vi "myDAQ Errors.vi"(8 "error in (no error)":errorcluster) -> (0 "error out":errorcluster)   [LabVIEW 2012]
doc: "This VI is designed to handel common myDAQ errors and give more useful specific error dialogs. It also finds a control names \"Stop\" in the calling VI and toggels it true to stop the VI."
uses:
  <vilib>/regexp/Match Regular Expression.xnode
panel:
  out "call chain":string[](array[string])
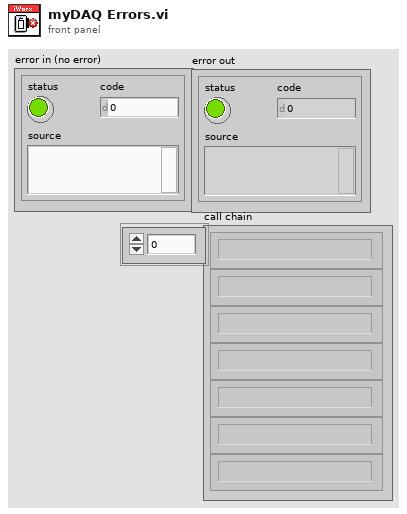
[diagram p1: front panel]
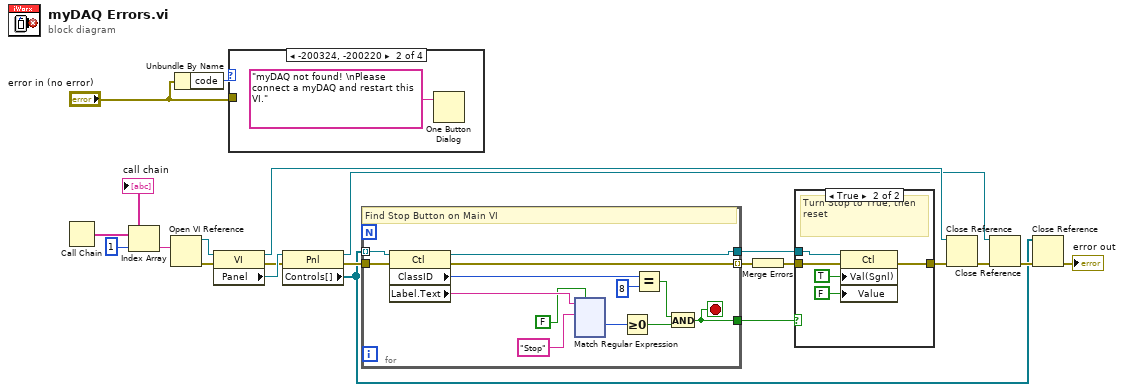
[diagram p0: block diagram]
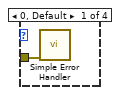
[diagram p3: hidden frame]
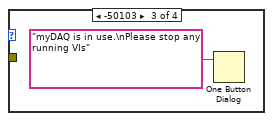
[diagram p4: hidden frame]
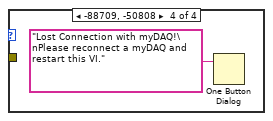
[diagram p5: hidden frame]
diagram:
  n1 = Call Chain() -> (call chain=w20:string[])
  "call chain" <- w20
  n2 = Index Array(array=w20, index=1) -> (element=w18:string)
  n3 = Open VI Reference(vi path=w18) -> (vi reference=w17:refnum<vi>, error out=w16:errorcluster)  [unwired: 5 in]
  n4 = Unbundle By Name("error in (no error)") -> ("code"=w21:i32)
  n5 = property class="VI"(reference=w17, error in=w16) -> (reference out=w8:refnum<vi>, error out=w11:errorcluster, "Panel"=w15:refnum<vi>)
  n6 = case shown="-200324, -200220" w21 {
    tunnel: "error in (no error)" -> [w22 _ _ _]
    frame 0, Default {
      n7 = call <vilib>:"Simple Error Handler.vi"("error in (no error)"=w22) -> ()  [unwired: 4 in, 5 out]
    }
    frame -200324, -200220 {
      n8 = One Button Dialog(message="myDAQ not found! \nPlease connect a myDAQ and restart this VI.") -> ()  [unwired: 1 in, 1 out]
    }
    frame -50103 {
      n9 = One Button Dialog(message="myDAQ is in use.\nPlease stop any running VIs") -> ()  [unwired: 1 in, 1 out]
    }
    frame -88709, -50808 {
      n10 = One Button Dialog(message="Lost Connection with myDAQ!\nPlease reconnect a myDAQ and restart this VI.") -> ()  [unwired: 1 in, 1 out]
    }
  }
  n11 = property class="Pnl"(reference=w15, error in=w11) -> (reference out=w5:refnum<vi>, error out=w12:errorcluster, "Controls[]"=w3:refnum<vi>[])
  n12 = for {
    tunnel: w3 -> [w38] mode=indexing
    tunnel: [w34] -> w14
    tunnel: [w33] -> w13
    tunnel: [w32] -> w10 mode=indexing
    tunnel: w12 -> [w31]
    stop <- w33 stop-if-true
    # "Find Stop Button on Main VI"
    n13 = property class="Ctl"(reference=w38, error in=w31) -> (reference out=w34:refnum<vi>, error out=w32:errorcluster, "ClassID"=w37:u32, "Label.Text"=w30:string)
    n14 = xnode "Match Regular Expression"("input string"=w30, "regular expression"="Stop" ("y"), "ignore case? (F)"=FALSE) -> ("offset past match"=w27:i32)  [unwired: 3 in, 4 out]
    n15 = Greater Or Equal To 0?(x=w27) -> (x >= 0?=w26:bool)
    n16 = Equal?(x=w37, y=u32 8) -> (x = y?=w35:bool)
    n17 = And(x=w35, y=w26) -> (x .and. y?=w33:bool)
  }
  n18 = Merge Errors(w10) -> (w9:errorcluster)
  n19 = case shown="True" w13 {
    tunnel: w14 -> [_ w155]
    tunnel: w9 -> [w150 w153]
    tunnel: [w150 w151] -> w7
    frame False {
      # "Do nothing"
    }
    frame True {
      # "Turn Stop to True, then reset"
      n20 = property class="Ctl"(reference=w155, error in=w153, "Val(Sgnl)"=TRUE, "Value"=FALSE) -> (error out=w151:errorcluster)  [unwired: 1 out]
    }
  }
  n21 = Close Reference(reference=w8, error in (no error)=w7) -> (error out=w6:errorcluster)
  n22 = Close Reference(reference=w5, error in (no error)=w6) -> (error out=w4:errorcluster)
  n23 = Close Reference(reference=w3, error in (no error)=w4) -> (error out=→"error out":errorcluster)
